vi "test Deployment.vi"(8 "error in (no error)":errorcluster, 11 "TestCase in":refnum<class "Routing and Faulting System Tests.lvclass">) -> (0 "error out":errorcluster, 3 "TestCase out":refnum<class "Routing and Faulting System Tests.lvclass">)   [LabVIEW 2017, in "Routing and Faulting System Tests.lvclass"]
uses:
  Routing and Faulting System Tests.lvclass
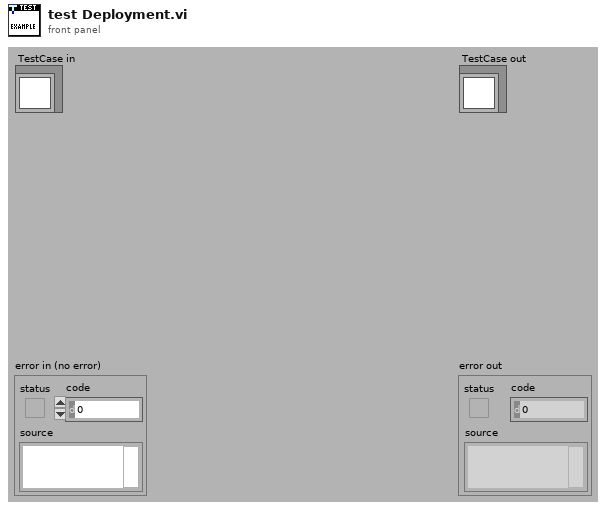
[diagram p1: front panel]
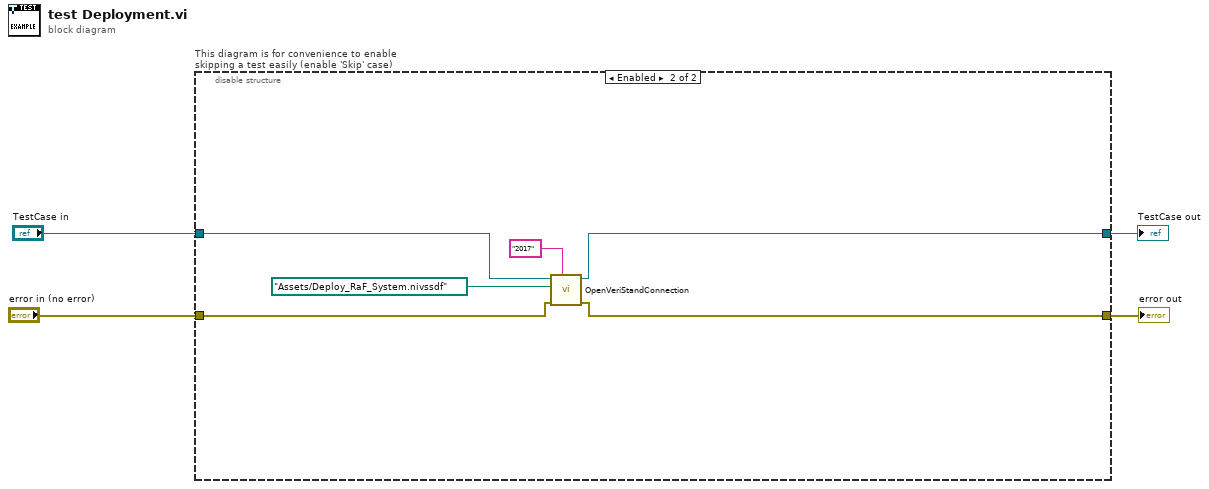
[diagram p0: block diagram]
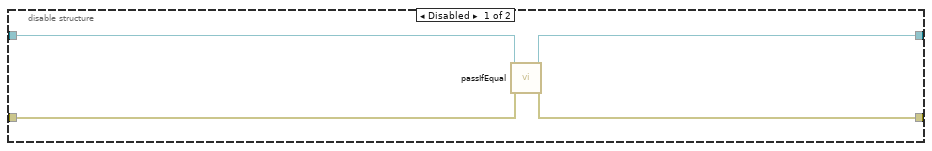
[diagram p2: hidden frame]
diagram:
  n1 = disable-structure "This diagram is for convenience to enable skipping a test easily (enable 'Skip' case)" shown="Enabled" {
    disable-tunnel: "TestCase in" -> [w8 w12]
    disable-tunnel: [w7 w11] -> w1
    disable-tunnel: [w6 w9] -> w3
    disable-tunnel: "error in (no error)" -> [w5 w10]
    frame Disabled {
      n2 = call-dynamic "passIfEqual.vi"("error in (no error)"=w5, "TestCase in"=w8) -> ("error out"=w6:errorcluster, "TestCase out"=w7:refnum<class "Routing and Faulting System Tests.lvclass">)  [unwired: 8 in]
    }
    frame Enabled {
      n3 = call-dynamic "OpenVeriStandConnection.vi"("Minimum VeriStand Version (2015)"="2017", "error in (no error)"=w10, "System Definition File"=path "Assets/Deploy_RaF_System.nivssdf", "VeriStand Test Case in"=w12) -> ("error out"=w9:errorcluster, "VeriStand Test Case out"=w11:refnum<class "Routing and Faulting System Tests.lvclass">)  [unwired: 5 in, 1 out]
    }
  }
  "error out" <- w3
  "TestCase out" <- w1
